vi "action - GitRepo Show Current Branch.vi"(8 "error in (no error)":errorcluster, 11 "Path":path) -> (3 "f":string)   [LabVIEW 2019]
uses:
  <vilib>/Hampel Software Engineering/Git API/Git API/GIT-api.lvclass/GIT-api.ctl
  <vilib>/Hampel Software Engineering/Git API/Git API/Accessors/GIT-Set Working Dir.vi
  <vilib>/Hampel Software Engineering/Git API/Git API/GIT-api.lvclass
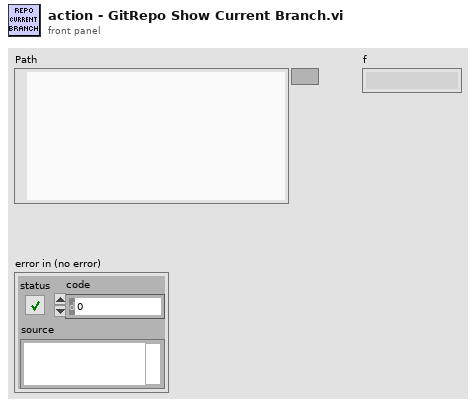
[diagram p1: front panel]
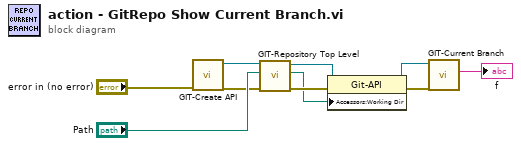
[diagram p0: block diagram]
diagram:
  n1 = call <vilib>:"GIT-Create API.vi"("error in"="error in (no error)") -> ("error out"=w3:errorcluster, "git-api out"=w5:refnum<class "GIT-api.lvclass">)  [unwired: 9 in]
  n2 = call <vilib>:"GIT-Repository Top Level.vi"("error in"=w3, "Current Path"="Path", "git-api in"=w5) -> ("error out"=w10:errorcluster, "Repo Top Level Path"=w8:path, "git-api out"=w9:refnum<class "GIT-api.lvclass">)  [unwired: 6 in]
  n3 = property class="Git-API"(reference=w9, error in=w10, "Accessors:Working Dir"=w8) -> (reference out=w7:refnum<class "GIT-api.lvclass">, error out=w6:errorcluster)
  n4 = call <vilib>:"GIT-Current Branch.vi"("error in"=w6, "git-api in"=w7) -> ("current branch"=→"f":string)  [unwired: 7 in, 2 out]
